vi "Application_CleanUp.vi"(8 "ErrorIn":errorcluster) -> (0 "ErrorOut":errorcluster)   [LabVIEW 2021, in "Application.lvclass"]
uses:
  Application.lvclass
  Application.lvclass/Application.ctl
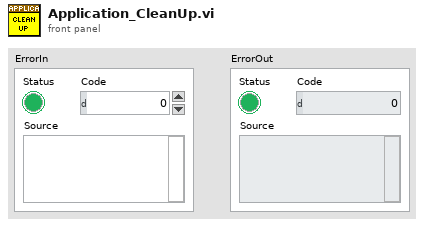
[diagram p1: front panel]
types:
  T1 = typedef "Application.lvclass/ObjectAttributes.ctl" = cluster{"Objects":variant, "BasePath":path, "Application":refnum<class "Application.lvclass">}
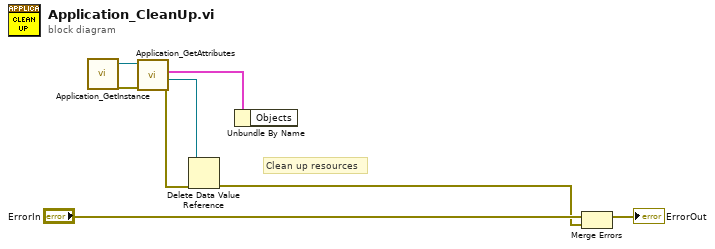
[diagram p0: block diagram]
diagram:
  # "Clean up resources"
  n1 = call "Application_GetInstance.vi"() -> ("ErrorOut"=w7:errorcluster, "ReferenceOut"=w2:refnum<class "Application.lvclass">)  [unwired: 7 in, 3 out]
  n2 = call "Application_GetAttributes.vi"("ErrorIn"=w7, "ReferenceIn"=w2) -> ("ErrorOut"=w6:errorcluster, "DataRef"=w1:refnum<data-value>, "Data"=w3:T1)  [unwired: 6 in, 1 out]
  n3 = Delete Data Value Reference(data value reference=w1, error in=w6) -> (error out=w4:errorcluster)  [unwired: 1 out]
  n4 = Unbundle By Name(w3) -> ()  [unwired: 1 out]
  n5 = Merge Errors("ErrorIn", w4) -> (→"ErrorOut":errorcluster)
